vi "Read Config v1.2.vi"(8 "error in":errorcluster, 11 "file path":path) -> (0 "error out":errorcluster, 2 "All Para":cluster{"Auto Para":T1, "General Para 2":T2}={"Auto Para"={"Agitator Delays"=[250, 600], "TF Delays"=[400, 800, 2, 8000], "Insertion Delays"=[100, 400], "Cutting Delays"=[150, 250, 50], "PF Delays"=[300, 8000], "Measur. Delays"=[200.0, 188.9, 1.0], "Reject Delays"=[500], "BF Delays"=[1000, 1000], "P&P Delays"=[1000]}, "General Para 2"={"Max. Cons."=5.0, "Offset 1"=0.0, "Offset 2"=0.0, "Offset 3"=0.0, "Offset 4"=-0.6, "OutputPause"=500.0, "RejectPause"=500.0, "IndexTimeout"=0.0}} {"General Para 2"."Offset 4" format="%.2f"; "General Para 2"."Offset 3" format="%.2f"; "General Para 2"."Offset 2" format="%.2f"; "General Para 2"."Offset 1" format="%.2f"}, 3 "file path out":path, 5 "password":string)   [LabVIEW 2021]
doc: "v1.0:\nRead 2WR Motor Bencg or not."
uses:
  RT/Controls/Auto Delays.ctl
  Controls/General Para.ctl
  <vilib>/Utility/config.llb/Read Key (Double).vi
  <vilib>/Utility/config.llb/Read Key (String).vi
  <vilib>/Utility/config.llb/NI_LVConfig.lvlib
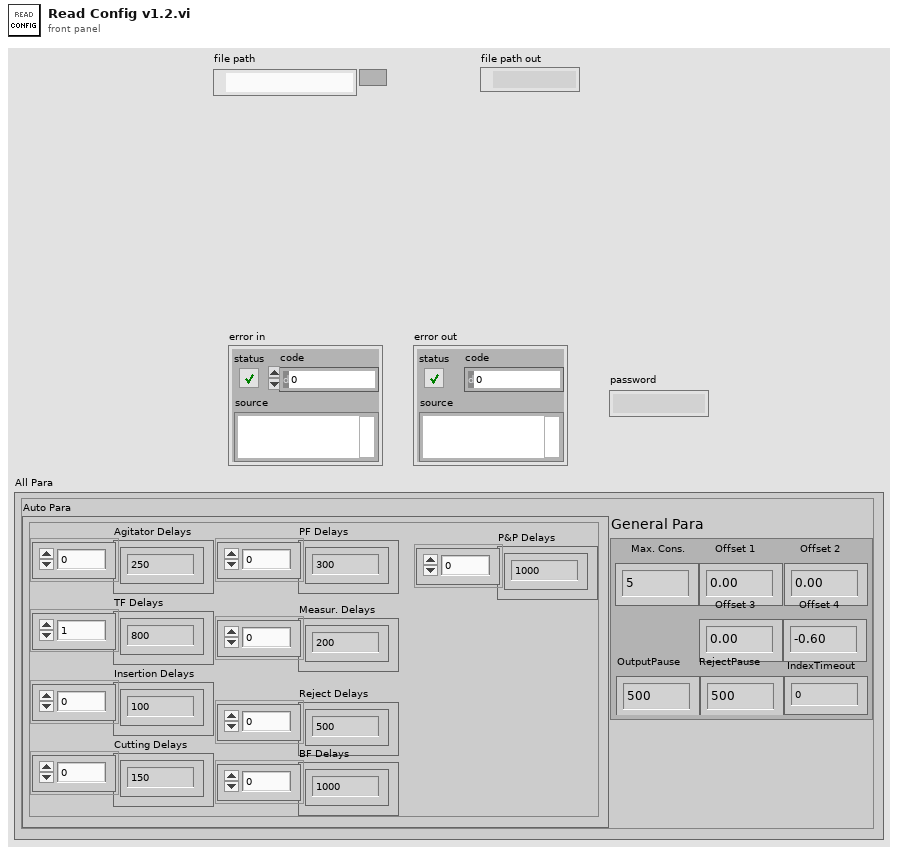
[diagram p1: front panel]
types:
  T1 = typedef "Auto Delays.ctl" = cluster{"Agitator Delays":u32[], "TF Delays":u32[], "Insertion Delays":u32[], "Cutting Delays":u32[], "PF Delays":u32[], "Measur. Delays":dbl[], "Reject Delays":u32[], "BF Delays":u32[], "P&P Delays":u32[]}
  T2 = typedef "General Para.ctl" = cluster{"Max. Cons.":dbl, "Offset 1":dbl, "Offset 2":dbl, "Offset 3":dbl, "Offset 4":dbl, "OutputPause":dbl, "RejectPause":dbl, "IndexTimeout":dbl}
  T3 = typedef "NI_LVConfig.lvlib/Config Data RefNum.ctl" = refnum<k1>
  T4 = cluster{"[0]":dbl, "[1]":dbl, "[2]":dbl, "[3]":dbl, "[4]":dbl, "[5]":dbl, "[6]":dbl, "[7]":dbl}
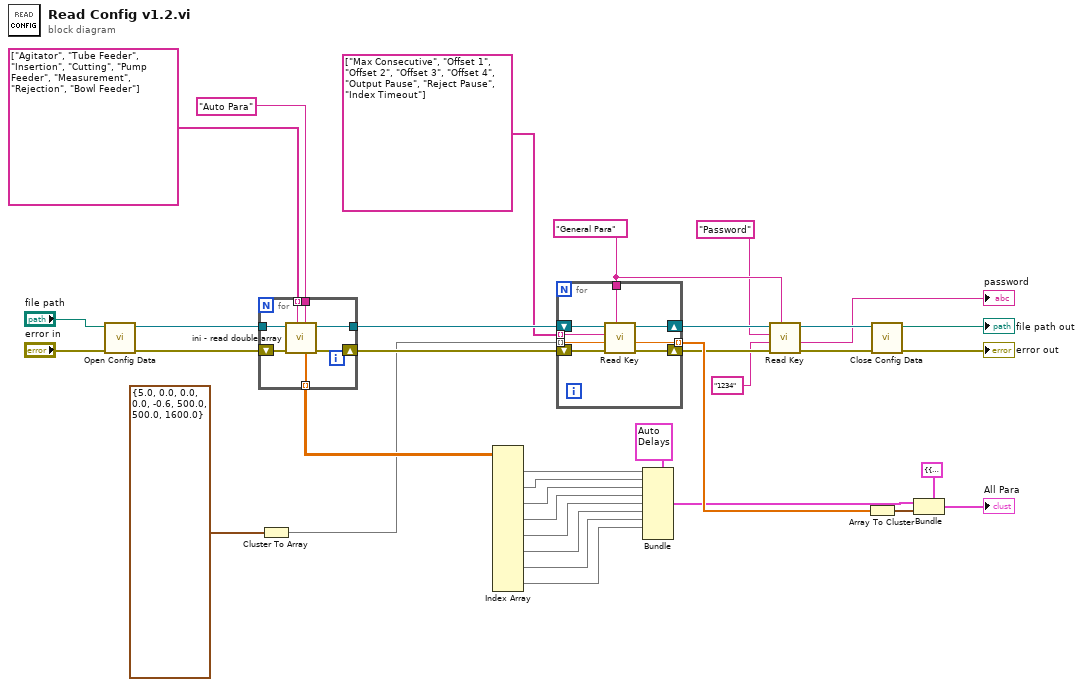
[diagram p0: block diagram]
diagram:
  w6 = "General Para" ("section")
  n1 = call <vilib>:"Open Config Data.vi"("error in (no error)"="error in", "configuration file path"="file path") -> ("error out"=w27:errorcluster, "refnum"=w28:T3)  [unwired: 7 in, 1 out]
  n2 = for {
    tunnel: w28 -> [w43]
    tunnel: "Auto Para" ("section") -> [w39]
    tunnel: string[] ["Agitator", "Tube Feeder", "Insertion", "Cutting", "Pump Feeder", "Measurement", "Rejection", "Bowl Feeder"] -> [w38] mode=indexing
    tunnel: [w40] -> w31
    shift-right: [w41] -> w30
    shift-left: w27 -> [w42]
    tunnel: [w37] -> w21 mode=indexing
    n3 = call "ini - read double array.vi"("section"=w39, "key"=w38, "error in"=w42, "refnum in"=w43) -> ("error out"=w41:errorcluster, "refnum out"=w40:T3, "double array"=w37:dbl[])  [unwired: 5 in]
  }
  n4 = Cluster To Array(cluster=T2 {"Max. Cons."=5.0, "Offset 1"=0.0, "Offset 2"=0.0, "Offset 3"=0.0, "Offset 4"=-0.6, "OutputPause"=500.0, "RejectPause"=500.0, "IndexTimeout"=1600.0} ("General Para 2")) -> (array=w1:dbl[])
  n5 = Index Array(array=w21) -> (element #1=w20:dbl[], element #2=w19:dbl[], element #3=w18:dbl[], element #4=w17:dbl[], element #5=w16:dbl[], element #6=w15:dbl[], element #7=w14:dbl[], element #8=w13:dbl[])  [unwired: 16 in]
  n6 = for {
    tunnel: w6 -> [w49]
    shift-right: [w51] -> w8
    shift-left: w31 -> [w48]
    shift-right: [w50] -> w10
    shift-left: w30 -> [w47]
    tunnel: string[] ["Max Consecutive", "Offset 1", "Offset 2", "Offset 3", "Offset 4", "Output Pause", "Reject Pause", "Index Timeout"] -> [w46] mode=indexing
    tunnel: [w45] -> w23 mode=indexing
    tunnel: w1 -> [w44] mode=indexing
    n7 = call-poly <vilib>:"Read Key.vi"("section"=w49, "error in (no error)"=w47, "default value"=w44, "key"=w46, "refnum"=w48) -> ("error out"=w50:errorcluster, "value"=w45:dbl, "refnum out"=w51:T3)  [unwired: 3 in, 1 out]
  }
  n8 = Bundle(cluster=T1 {"Agitator Delays"=[250, 600], "TF Delays"=[400, 800, 2, 8000], "Insertion Delays"=[100, 400], "Cutting Delays"=[150, 250, 50], "PF Delays"=[300, 8000], "Measur. Delays"=[200.0, 188.9, 1.0], "Reject Delays"=[500], "BF Delays"=[1000, 1000], "P&P Delays"=[1000]} ("Auto Para"), "Agitator Delays"=w20, "TF Delays"=w19, "Insertion Delays"=w18, "Cutting Delays"=w17, "PF Delays"=w16, "Measur. Delays"=w15, "Reject Delays"=w14, "BF Delays"=w13) -> (w12:T1)  [unwired: 1 in]
  n9 = call-poly <vilib>:"Read Key.vi"("section"=w6, "error in (no error)"=w10, "default value"="1234", "key"="Password", "refnum"=w8) -> ("error out"=w9:errorcluster, "value"=→"password":string, "refnum out"=w7:T3)  [unwired: 3 in, 1 out]
  n10 = Array To Cluster(array=w23) -> (cluster=w24:T4)
  n11 = call <vilib>:"Close Config Data.vi"("error in (no error)"=w9, "refnum"=w7) -> ("error out"=→"error out":errorcluster, "file path"=→"file path out":path)  [unwired: 8 in]
  n12 = Bundle(cluster=cluster{"Auto Para":T1, "General Para 2":T2} {"Auto Para"={"Agitator Delays"=[250, 600], "TF Delays"=[400, 800, 2, 8000], "Insertion Delays"=[100, 400], "Cutting Delays"=[150, 250, 50], "PF Delays"=[300, 8000], "Measur. Delays"=[200.0, 188.9, 1.0], "Reject Delays"=[500], "BF Delays"=[1000, 1000], "P&P Delays"=[1000]}, "General Para 2"={"Max. Cons."=5.0, "Offset 1"=0.0, "Offset 2"=0.0, "Offset 3"=0.0, "Offset 4"=-0.6, "OutputPause"=500.0, "RejectPause"=500.0, "IndexTimeout"=0.0}} ("All Para"), "Auto Para"=w12, "General Para 2"=w24) -> (→"All Para":cluster{"Auto Para":T1, "General Para 2":T2})
